vi "NI Datatype to Generic DataType.vi"(11 "NI Datatype":T1) -> (3 "Generic Datatype":T2=enum."Bool")   [LabVIEW 2021, in "DataTypes_CIF_U.lvlib"]
doc: "Convert NI datatypes into generic datatypes. This is useful when flattening the datatypes or providing them dynamically into C functions."
uses:
  DataTypes_CIF_U.lvlib
  Typedef/Generic Datatypes.ctl
  <vilib>/Utility/Data Type/Type Definitions/Data Type.ctl
  <vilib>/Utility/Data Type/NI_Data Type.lvlib
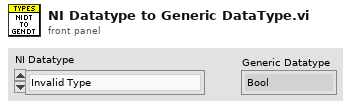
[diagram p1: front panel]
types:
  T1 = typedef "NI_Data Type.lvlib/Data Type.ctl" = enum8{"Invalid Type", "Void", "I8", "I16", "I32", "I64", "U8", "U16", "U32", "U64", "Single Float", "Double Float", "Extended Float", "Single Complex", "Double Complex", "Extended Complex", "Enum U8", "Enum U16", "Enum U32", "Enum U64", "Single Float With Unit", "Double Float With Unit", "Extended Float With Unit", "Single Complex with Unit", "Double Complex with Unit", "Extended Complex with Unit", "Boolean", "String", "Path", "Picture", "Tag", "Array", "Cluster", "Variant", "LV Variant", "Waveform", "Timestamp", "Digital Waveform", "Digital Data", "ExpressData", "Refnum", "External Data", "VI", "Poly VI", "LabVIEW Class Instance", "Fixed Point", "Set Collection", "Map Collection"}
  T2 = typedef "DataTypes_CIF_U.lvlib/Generic Datatypes.ctl" = enum16{"Invalid", "Bool", "U8", "I8", "U16", "I16", "U32", "I32", "U64", "I64", "Single Float", "Double Float", "String"}
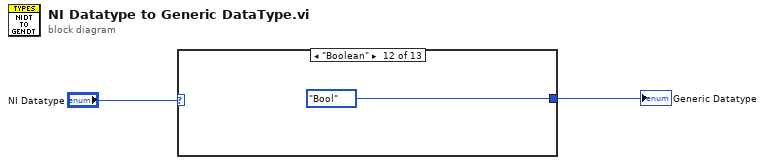
[diagram p0: block diagram]
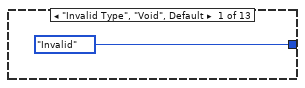
[diagram p2: hidden frame]
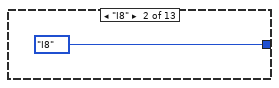
[diagram p3: hidden frame]
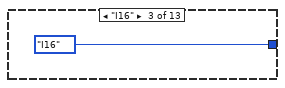
[diagram p4: hidden frame]
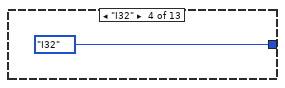
[diagram p5: hidden frame]
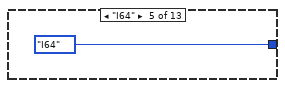
[diagram p6: hidden frame]
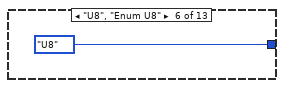
[diagram p7: hidden frame]
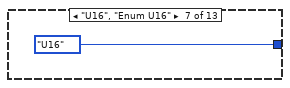
[diagram p8: hidden frame]
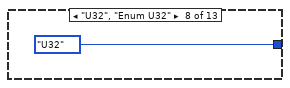
[diagram p9: hidden frame]
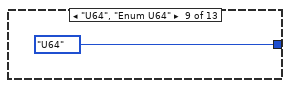
[diagram p10: hidden frame]
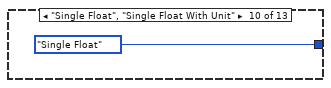
[diagram p11: hidden frame]
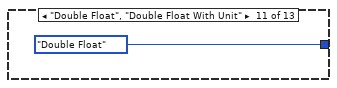
[diagram p12: hidden frame]
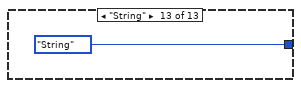
[diagram p13: hidden frame]
diagram:
  n1 = case shown="\"Boolean\"" "NI Datatype" {
    tunnel: [Generic_Datatypes."Invalid" ("Generic Datatype") Generic_Datatypes."I8" ("Generic Datatype") Generic_Datatypes."I16" ("Generic Datatype") Generic_Datatypes."I32" ("Generic Datatype") Generic_Datatypes."I64" ("Generic Datatype") Generic_Datatypes."U8" ("Generic Datatype") Generic_Datatypes."U16" ("Generic Datatype") Generic_Datatypes."U32" ("Generic Datatype") Generic_Datatypes."U64" ("Generic Datatype") Generic_Datatypes."Single Float" ("Generic Datatype") Generic_Datatypes."Double Float" ("Generic Datatype") Generic_Datatypes."Bool" ("Generic Datatype") Generic_Datatypes."String" ("Generic Datatype")] -> w2
    frame "Invalid Type", "Void", Default {
    }
    frame "I8" {
    }
    frame "I16" {
    }
    frame "I32" {
    }
    frame "I64" {
    }
    frame "U8", "Enum U8" {
    }
    frame "U16", "Enum U16" {
    }
    frame "U32", "Enum U32" {
    }
    frame "U64", "Enum U64" {
    }
    frame "Single Float", "Single Float With Unit" {
    }
    frame "Double Float", "Double Float With Unit" {
    }
    frame "Boolean" {
    }
    frame "String" {
    }
  }
  "Generic Datatype" <- w2
